vi "MQTT_SSL_Publish.vi"(6 "Message ID":u16=10 format="%x", 7 "Publish Meta":cluster{"QoS":T2, "Retain":T3, "DUP":T4}, 8 "error in (no error)":errorcluster, 9 "Message to be published":string=" Message", 10 "Topic":string="a/b", 11 "SSL_Connection":T1) -> (0 "error out":errorcluster, 3 "SSL_Connection":T1)   [LabVIEW 2018, in "AWS_IoT.lvlib"]
doc: "This VI publishes a message to a registered topic.\n\n© 2015 - daq.io, LLC - Peter Adelhardt"
uses:
  AWS_IoT.lvlib
  Controls/QoS.ctl
  Controls/Retain_Flag.ctl
  Controls/DUP_Flag.ctl
  Controls/SSL_Connection.ctl
  Controls/MessageType.ctl
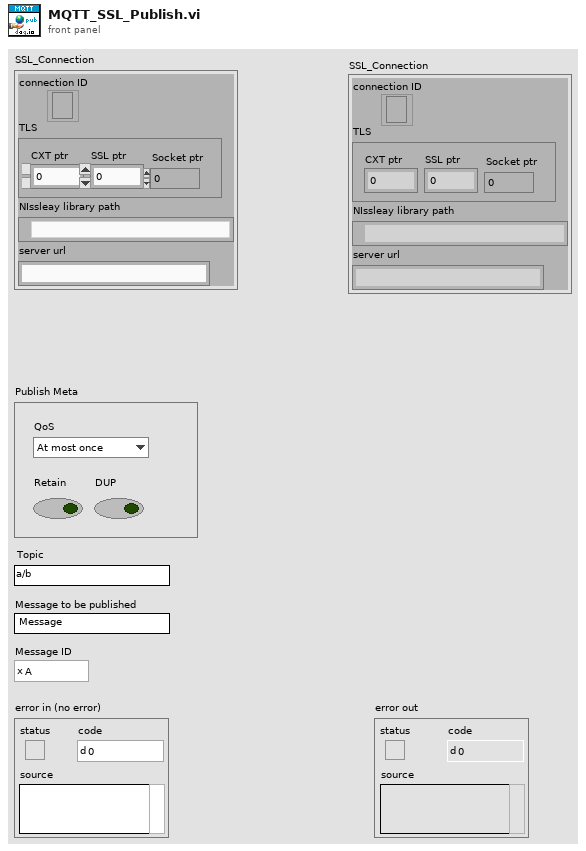
[diagram p1: front panel]
types:
  T1 = typedef "AWS_IoT.lvlib/SSL_Connection.ctl" = cluster{"connection ID":refnum<k5>, "TLS":cluster{"CXT ptr":i32, "SSL ptr":i32, "Socket ptr":i32}, "NIssleay library path":path, "server url":string}
  T2 = typedef "AWS_IoT.lvlib/QoS.ctl" = enum8{"At most once", "At least once", "Exactly once", "Reserved"}
  T3 = typedef "AWS_IoT.lvlib/Retain_Flag.ctl" = bool
  T4 = typedef "AWS_IoT.lvlib/DUP_Flag.ctl" = bool
  T5 = typedef "AWS_IoT.lvlib/MessageType.ctl" = enum32{"Reserved", "CONNECT", "CONNACK", "PUBLISH", "PUBACK", "PUBREC", "PUBREL", "PUBCOMP", "SUBSCRIBE", "SUBACK", "UNSUBSCRIBE", "UNSUBACK", "PINGREQ", "PINGRESP", "DISCONNECT", "Reserved2"}
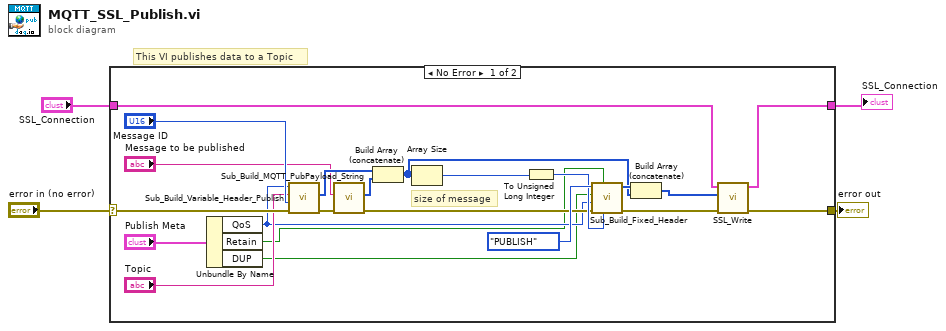
[diagram p0: block diagram]
diagram:
  # "This VI publishes data to a Topic"
  n1 = case shown="No Error" "error in (no error)" {
    selector: "error in (no error)" -> [w25 w28]
    tunnel: [w8 w28] -> w3
    tunnel: "SSL_Connection" -> [w6 w27]
    tunnel: [w5 w27] -> w1
    frame No Error {
      # "size of message"
      n2 = Unbundle By Name("Publish Meta") -> ("QoS"=w12:T2, "Retain"=w11:T3, "DUP"=w10:T4)
      n3 = call "Sub_Build_Variable_Header_Publish.vi"("error in (no error)"=w25, "Message ID"="Message ID", "Topic Name"="Topic", "QoS"=w12) -> ("error out"=w21:errorcluster, "Variable Header"=w19:u8[])  [unwired: 6 in]
      n4 = call "Sub_Build_MQTT_PubPayload_String.vi"("error in (no error)"=w21, "String to be encoded"="Message to be published") -> ("error out"=w20:errorcluster, "UTF8 Byte Array"=w18:u8[])  [unwired: 8 in]
      n5 = Build Array (concatenate)(w19, w18) -> (w16:u8[])
      n6 = Array Size(array=w16) -> (size(s)=w22:i32)
      n7 = To Unsigned Long Integer(number=w22) -> (unsigned 32bit integer=w23:u32)
      n8 = call "Sub_Build_Fixed_Header.vi"("Remaining Length"=w23, "Retain"=w11, "error in (no error)"=w20, "QoS"=w12, "DUP"=w10, "MessageType"=MessageType."PUBLISH") -> ("error out"=w9:errorcluster, "Fixed Header"=w17:u8[])  [unwired: 4 in]
      n9 = Build Array (concatenate)(w17, w16) -> (w7:u8[])
      n10 = call "SSL_Write.vi"("error in (no error)"=w9, "data in"=w7, "SSL_Connection"=w6) -> ("error out"=w8:errorcluster, "SSL_Connection"=w5:T1)  [unwired: 7 in]
    }
    frame Error {
    }
  }
  "error out" <- w3
  "SSL_Connection" <- w1
